vi "WRITE FGV.vi"(7 "Enum":T1=enum."WRITE", 8 "error in (no error)":errorcluster, 10 "data":dbl[](array[numeric]) format="%.2f", 11 "signal list":refnum<k21>[](array[refnum])) -> (0 "error out":errorcluster, 2 "Array":dbl[](array[numeric]))   [LabVIEW 2018]
uses:
  FGV States.ctl
  <vilib>/xnet/xnet.llb/XNET Write (Signal Single-point).vi
  <vilib>/xnet/xnet.llb/XNET Create Session (Signal Input Single-point).vi
  <vilib>/xnet/xnet.llb/XNET Read (Signal Single-point).vi
  <vilib>/xnet/xnet.llb/XNET Create Session (Signal Output Single-point).vi
  <resource>/objmgr/xnet.rc
panel:
  out "data 2":dbl[](array[numeric]) caption="data" format="%.2f"
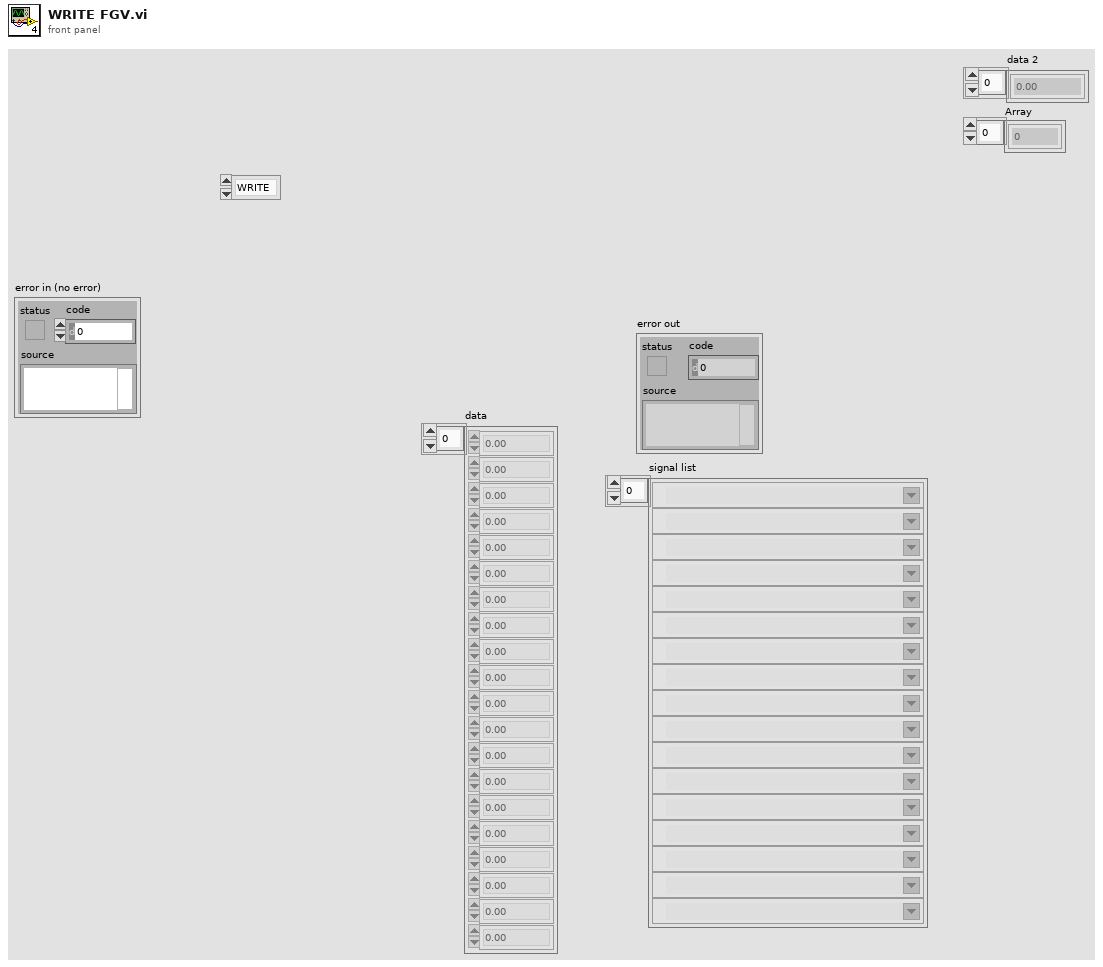
[diagram p1: front panel]
types:
  T1 = typedef "FGV States.ctl" = enum16{"OPEN", "READ", "CLOSE", "WRITE"}
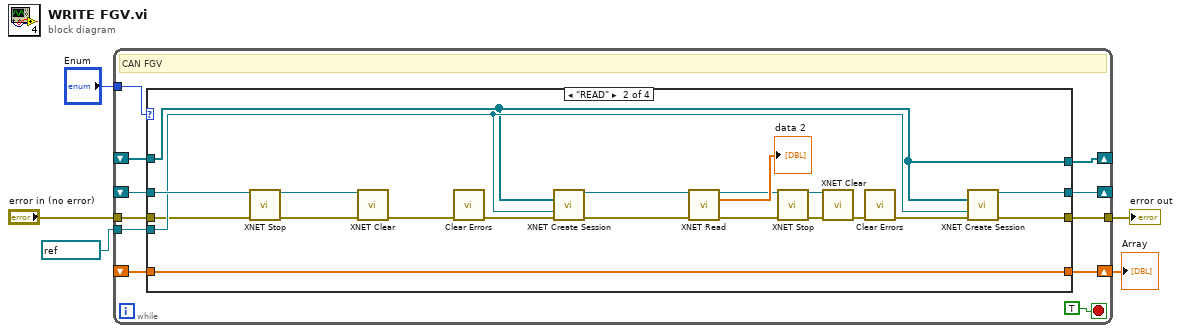
[diagram p0: block diagram]
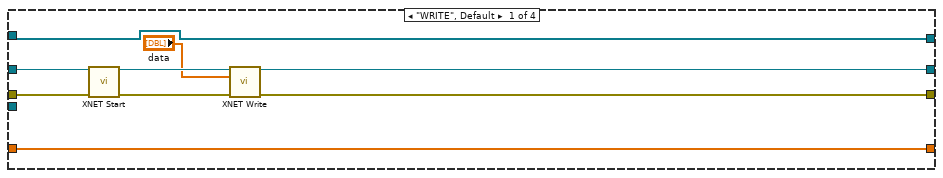
[diagram p2: hidden frame]
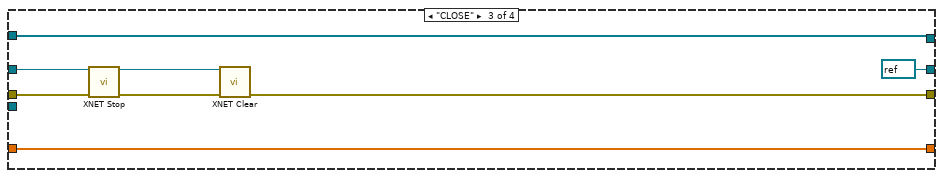
[diagram p3: hidden frame]
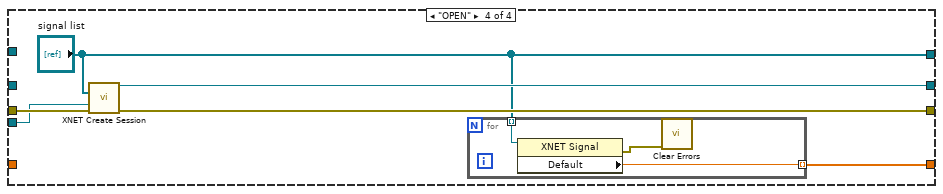
[diagram p4: hidden frame]
diagram:
  n1 = while {
    tunnel: "Enum" -> [w15]
    shift-right: [w14] -> _
    shift-left: _ -> [w13]
    tunnel: [w12] -> w3
    tunnel: "error in (no error)" -> [w11]
    tunnel: refnum<k21> "CAN1" ("Select Interface") -> [w9]
    shift-right: [w8] -> _
    shift-left: _ -> [w10]
    shift-right: [w7] -> w1
    shift-left: _ -> [w6]
    stop <- TRUE stop-if-true
    # "CAN FGV"
    n2 = case shown="\"READ\"" w15 {
      tunnel: [w24 w32 refnum<k21> refnum ("session out") w57] -> w14
      tunnel: w13 -> [w21 w42 w49 _]
      tunnel: [w25 w29 w50 w58] -> w12
      tunnel: w11 -> [w23 w28 w51 w59]
      tunnel: w10 -> [w18 w27 w47 _]
      tunnel: w9 -> [_ w31 _ w56]
      tunnel: [w18 w27 w47 "signal list"] -> w8
      tunnel: [w17 w26 w46 w54] -> w7
      tunnel: w6 -> [w17 w26 w46 _]
      frame "WRITE", Default {
        n3 = call <vilib>:"XNET Start.vi"("session in"=w21, "error in (no error)"=w23) -> ("session out"=w20:refnum<k21>, "error out"=w22:errorcluster)  [unwired: 12 in]
        n4 = call-poly <vilib>:"XNET Write.vi"("session in"=w20, "data"="data", "error in (no error)"=w22) -> ("session out"=w24:refnum<k21>, "error out"=w25:errorcluster)  [unwired: 11 in]
      }
      frame "READ" {
        n5 = call <vilib>:"XNET Stop.vi"("session in"=w42, "error in (no error)"=w28) -> ("session out"=w44:refnum<k21>, "error out"=w43:errorcluster)  [unwired: 12 in]
        n6 = call <vilib>:"XNET Clear.vi"("session in"=w44, "error in (no error)"=w43) -> ("error out"=w41:errorcluster)  [unwired: 13 in]
        n7 = call <vilib>:"Clear Errors.vi"("error in (no error)"=w41) -> ("error out"=w40:errorcluster)  [unwired: 5 in, 1 out]
        n8 = call-poly <vilib>:"XNET Create Session.vi"("signal list"=w27, "interface"=w31, "error in (no error)"=w40) -> ("session out"=w39:refnum<k21>, "error out"=w38:errorcluster)  [unwired: 11 out]
        n9 = call-poly <vilib>:"XNET Read.vi"("session in"=w39, "error in (no error)"=w38) -> ("session out"=w33:refnum<k21>, "data"=→"data 2":dbl[], "error out"=w36:errorcluster)  [unwired: 11 in]
        n10 = call <vilib>:"XNET Stop.vi"("session in"=w33, "error in (no error)"=w36) -> ("session out"=w34:refnum<k21>, "error out"=w37:errorcluster)  [unwired: 12 in]
        n11 = call <vilib>:"XNET Clear.vi"("session in"=w34, "error in (no error)"=w37) -> ("error out"=w35:errorcluster)  [unwired: 13 in]
        n12 = call <vilib>:"Clear Errors.vi"("error in (no error)"=w35) -> ("error out"=w30:errorcluster)  [unwired: 5 in, 1 out]
        n13 = call-poly <vilib>:"XNET Create Session.vi"("signal list"=w27, "interface"=w31, "error in (no error)"=w30) -> ("session out"=w32:refnum<k21>, "error out"=w29:errorcluster)  [unwired: 11 out]
      }
      frame "CLOSE" {
        n14 = call <vilib>:"XNET Stop.vi"("session in"=w49, "error in (no error)"=w51) -> ("session out"=w52:refnum<k21>, "error out"=w53:errorcluster)  [unwired: 12 in]
        n15 = call <vilib>:"XNET Clear.vi"("session in"=w52, "error in (no error)"=w53) -> ("error out"=w50:errorcluster)  [unwired: 13 in]
      }
      frame "OPEN" {
        n16 = call-poly <vilib>:"XNET Create Session.vi"("signal list"="signal list", "interface"=w56, "error in (no error)"=w59) -> ("session out"=w57:refnum<k21>, "error out"=w58:errorcluster)  [unwired: 11 out]
        n17 = for {
          tunnel: "signal list" -> [w62] mode=indexing
          tunnel: [w61] -> w54 mode=indexing
          n18 = property class="XNET Signal"(reference=w62) -> (error out=w60:errorcluster, "Default"=w61:dbl)  [unwired: 1 in, 1 out]
          n19 = call <vilib>:"Clear Errors.vi"("error in (no error)"=w60) -> ()  [unwired: 5 in, 2 out]
        }
      }
    }
  }
  "error out" <- w3
  "Array" <- w1
